vi "Grade Ranking Results.vi"(8 "Error in":errorcluster caption="Error in (no error)", 11 "VIAResult":T11 {"Test Config Data"."Test Ranking" items=["Low", "Normal", "High"]}) -> (0 "Error out":errorcluster, 3 "Stats by Ranking":T1)   [LabVIEW 2023, in "VIA Results Handling.lvlib"]
doc: "Takes in VIA Results and converts it into a Stats by Ranking."
uses:
  VIA Results Handling.lvlib
  <vilib>/addons/analyzer/_analyzerctrls.llb/VIAnCtl Results.ctl
  <vilib>/addons/analyzer/_analyzerctrls.llb/VIAnCtl ResultsData (index).ctl
  <vilib>/addons/analyzer/_analyzerctrls.llb/VIAnCtl ResultStatus.ctl
  <vilib>/addons/analyzer/_vianresshared.llb/VIAnRes Parsed Results Data (by VI).ctl
  <vilib>/addons/analyzer/_vianresshared.llb/VIAnRes Parsed Results Data (by Test).ctl
  <vilib>/addons/analyzer/_analyzerctrls.llb/VIAnCtl Test Config Data.ctl
  <vilib>/addons/analyzer/_analyzerctrls.llb/VIAnCtl TestRanking.ctl
  <vilib>/addons/analyzer/_analyzerctrls.llb/VIAnCtl Config Control Value.ctl
  Stats by Ranking.ctl
  Stats Cluster.ctl
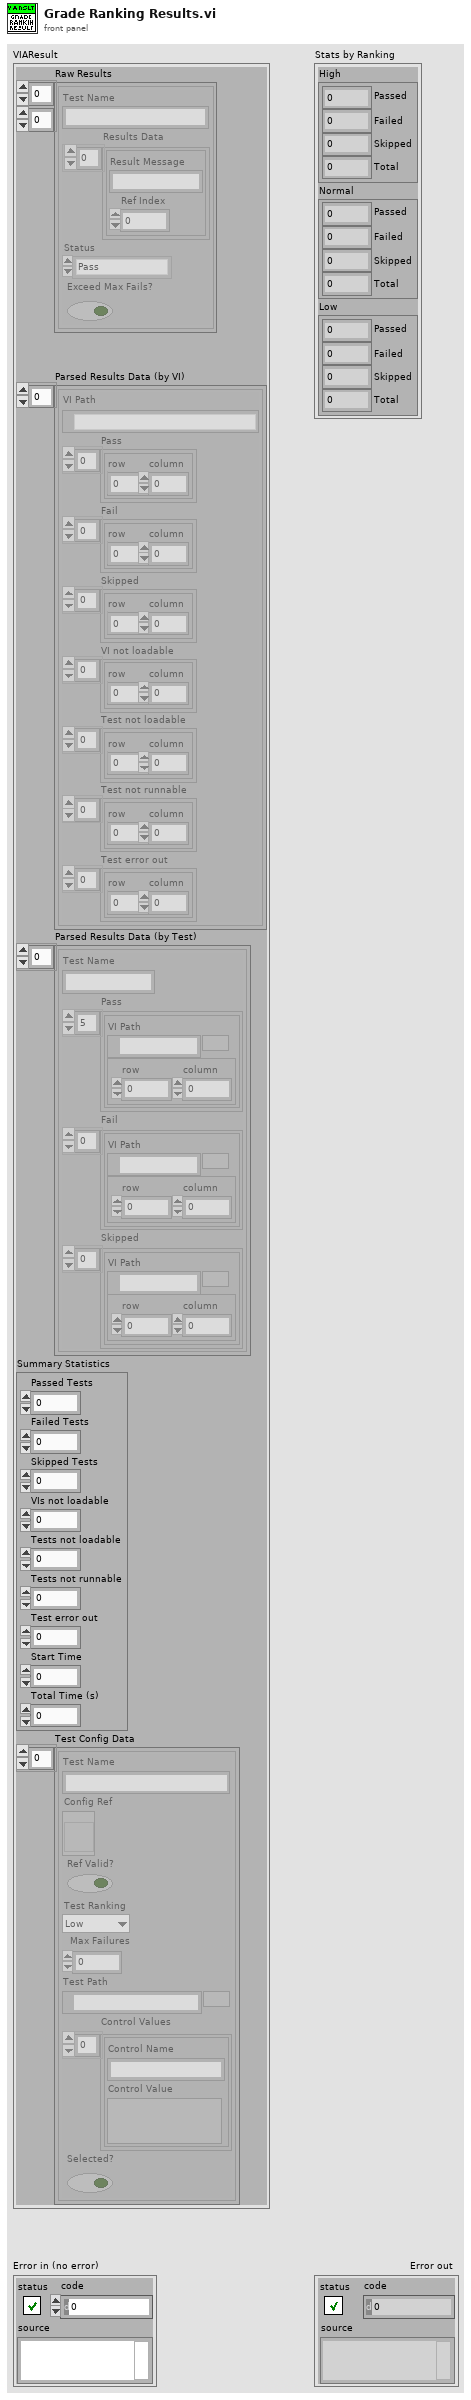
[diagram p1: front panel]
types:
  T1 = typedef "VIA Results Handling.lvlib/Stats by Ranking.ctl" = cluster{"High":T2, "Normal":T2, "Low":T2}
  T2 = typedef "VIA Results Handling.lvlib/Stats Cluster.ctl" = cluster{"Passed":i32, "Failed":i32, "Skipped":i32, "Total":i32}
  T3 = typedef "VIAnCtl Results.ctl" = cluster{"Test Name":string, "Results Data":T4[], "Status":T5, "Exceed Max Fails?":bool}
  T4 = typedef "VIAnCtl ResultsData (index).ctl" = cluster{"Result Message":string, "Ref Index":i32}
  T5 = typedef "VIAnCtl ResultStatus.ctl" = enum16{"Pass", "Fail", "Skipped", "VI not loadable", "Test not loadable", "Test not runnable", "Test error out"}
  T6 = typedef "VIAnRes Parsed Results Data (by VI).ctl" = cluster{"VI Path":path, "Pass":cluster{"row":i32, "column":i32}[], "Fail":cluster{"row":i32, "column":i32}[], "Skipped":cluster{"row":i32, "column":i32}[], "VI not loadable":cluster{"row":i32, "column":i32}[], "Test not loadable":cluster{"row":i32, "column":i32}[], "Test not runnable":cluster{"row":i32, "column":i32}[], "Test error out":cluster{"row":i32, "column":i32}[]}
  T7 = typedef "VIAnRes Parsed Results Data (by Test).ctl" = cluster{"Test Name":string, "Pass":cluster{"VI Path":path, "index":cluster{"row":i32, "column":i32}}[], "Fail":cluster{"VI Path":path, "index":cluster{"row":i32, "column":i32}}[], "Skipped":cluster{"VI Path":path, "index":cluster{"row":i32, "column":i32}}[]}
  T8 = typedef "VIAnCtl Test Config Data.ctl" = cluster{"Test Name":string, "Config Ref":refnum<vi>, "Ref Valid?":bool, "Test Ranking":T9, "Max Failures":u32, "Test Path":path, "Control Values":T10[], "Selected?":bool}
  T9 = typedef "VIAnCtl TestRanking.ctl" = u16
  T10 = typedef "VIAnCtl Config Control Value.ctl" = cluster{"Control Name":string, "Control Value":variant}
  T11 = cluster{"Raw Results":T3[][], "Parsed Results Data (by VI)":T6[], "Parsed Results Data (by Test)":T7[], "Summary Statistics":cluster{"Passed Tests":i32, "Failed Tests":i32, "Skipped Tests":i32, "VIs not loadable":i32, "Tests not loadable":i32, "Tests not runnable":i32, "Test error out":i32, "Start Time":u32, "Total Time (s)":dbl}, "Test Config Data":T8[]}
  T12 = typedef "VIA Results Handling.lvlib/Test Config Map.ctl" = map{string, T8}
  T13 = cluster{"VI Path":path, "index":cluster{"row":i32, "column":i32}}[]
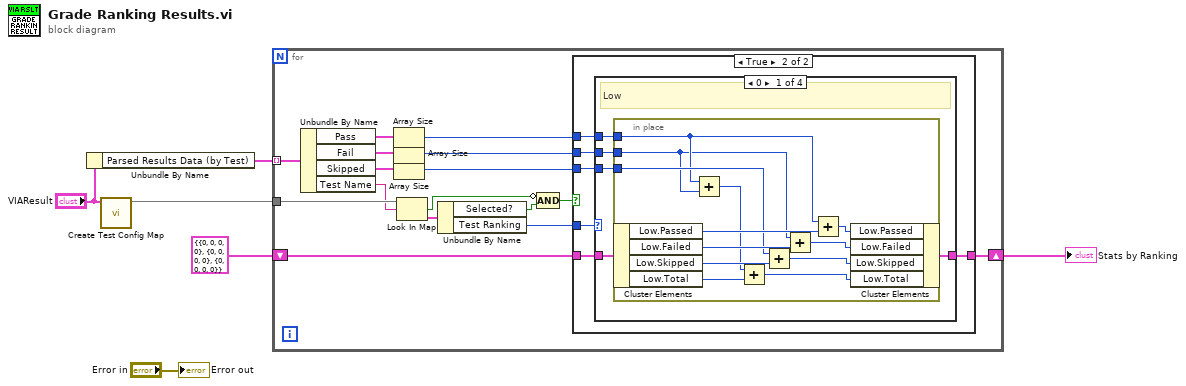
[diagram p0: block diagram]
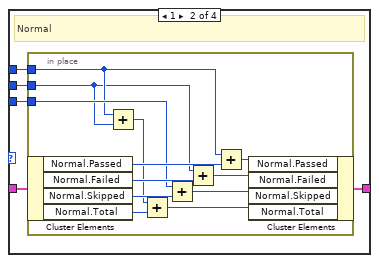
[diagram p3: hidden frame]
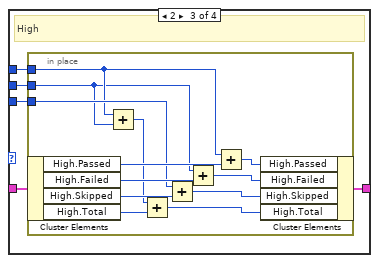
[diagram p4: hidden frame]
diagram:
  n1 = Unbundle By Name("VIAResult") -> ("Parsed Results Data (by Test)"=w4:T7[])
  n2 = call "Create Test Config Map.vi"("VIAResult"="VIAResult") -> ("Test Config Map"=w3:T12)  [unwired: 10 in]
  n3 = for {
    shift-right: [w11] -> w1
    shift-left: T1 {"High"={"Passed"=0, "Failed"=0, "Skipped"=0, "Total"=0}, "Normal"={"Passed"=0, "Failed"=0, "Skipped"=0, "Total"=0}, "Low"={"Passed"=0, "Failed"=0, "Skipped"=0, "Total"=0}} ("Stats by Ranking") -> [w12]
    tunnel: w4 -> [w22] mode=indexing
    tunnel: w3 -> [w18]
    n4 = Unbundle By Name(w22) -> ("Pass"=w21:T13, "Fail"=w20:T13, "Skipped"=w19:T13, "Test Name"=w17:string)
    n5 = Array Size(array=w21) -> (size(s)=w7:i32)
    n6 = Array Size(array=w20) -> (size(s)=w8:i32)
    n7 = Array Size(array=w19) -> (size(s)=w9:i32)
    n8 = Look In Map(map=w18, key=w17) -> (key not found?=w14:bool, value=w16:T8)  [unwired: 1 in]
    n9 = Unbundle By Name(w16) -> ("Selected?"=w15:bool, "Test Ranking"=w10:T9)
    n10 = Compound Arithmetic op=AND(invert w14, w15) -> (w13:bool)
    n11 = case shown="True" w13 {
      tunnel: w12 -> [w23 w27]
      tunnel: [w23 w28] -> w11
      tunnel: w10 -> [_ w29]
      tunnel: w9 -> [_ w26]
      tunnel: w8 -> [_ w25]
      tunnel: w7 -> [_ w24]
      frame False {
      }
      frame True {
        n12 = case shown="0" w29 {
          tunnel: [w30 w47 w64 w81] -> w28
          tunnel: w27 -> [w34 w51 w68 w81]
          tunnel: w26 -> [w33 w50 w67 _]
          tunnel: w25 -> [w32 w49 w66 _]
          tunnel: w24 -> [w31 w48 w65 _]
          frame 0 {
            # "Low"
            n13 = in-place {
              in-place-border: w33 -> [w42]
              in-place-border: w32 -> [w38]
              in-place-border: w31 -> [w39]
              n14 = in-place-cluster #1(w34) -> ("Low.Passed"=w46:i32, "Low.Failed"=w44:i32, "Low.Skipped"=w41:i32, "Low.Total"=w37:i32)
              n15 = Add(x=w39, y=w38) -> (x+y=w36:i32)
              n16 = Add(x=w36, y=w37) -> (x+y=w35:i32)
              n17 = Add(x=w42, y=w41) -> (x+y=w40:i32)
              n18 = Add(x=w38, y=w44) -> (x+y=w43:i32)
              n19 = Add(x=w39, y=w46) -> (x+y=w45:i32)
              n20 = in-place-cluster #1("Low.Passed"=w45, "Low.Failed"=w43, "Low.Skipped"=w40, "Low.Total"=w35) -> (w30:T1)
            }
          }
          frame 1 {
            # "Normal"
            n21 = in-place {
              in-place-border: w50 -> [w59]
              in-place-border: w49 -> [w55]
              in-place-border: w48 -> [w56]
              n22 = in-place-cluster #2(w51) -> ("Normal.Passed"=w63:i32, "Normal.Failed"=w61:i32, "Normal.Skipped"=w58:i32, "Normal.Total"=w54:i32)
              n23 = Add(x=w56, y=w55) -> (x+y=w53:i32)
              n24 = Add(x=w53, y=w54) -> (x+y=w52:i32)
              n25 = Add(x=w59, y=w58) -> (x+y=w57:i32)
              n26 = Add(x=w55, y=w61) -> (x+y=w60:i32)
              n27 = Add(x=w56, y=w63) -> (x+y=w62:i32)
              n28 = in-place-cluster #2("Normal.Passed"=w62, "Normal.Failed"=w60, "Normal.Skipped"=w57, "Normal.Total"=w52) -> (w47:T1)
            }
          }
          frame 2 {
            # "High"
            n29 = in-place {
              in-place-border: w67 -> [w76]
              in-place-border: w66 -> [w72]
              in-place-border: w65 -> [w73]
              n30 = in-place-cluster #3(w68) -> ("High.Passed"=w80:i32, "High.Failed"=w78:i32, "High.Skipped"=w75:i32, "High.Total"=w71:i32)
              n31 = Add(x=w73, y=w72) -> (x+y=w70:i32)
              n32 = Add(x=w70, y=w71) -> (x+y=w69:i32)
              n33 = Add(x=w76, y=w75) -> (x+y=w74:i32)
              n34 = Add(x=w72, y=w78) -> (x+y=w77:i32)
              n35 = Add(x=w73, y=w80) -> (x+y=w79:i32)
              n36 = in-place-cluster #3("High.Passed"=w79, "High.Failed"=w77, "High.Skipped"=w74, "High.Total"=w69) -> (w64:T1)
            }
          }
          frame Default {
          }
        }
      }
    }
  }
  "Stats by Ranking" <- w1
  "Error out" <- "Error in"
